vi "Read Time.vi"(8 "error in (no error)":errorcluster, 11 "ControlDragStartingMsg In":refnum<class "ControlDragStartingMsg.lvclass">) -> (0 "error out":errorcluster, 2 "Time":u32, 3 "ControlDragStartingMsg Out":refnum<class "ControlDragStartingMsg.lvclass">)   [LabVIEW 2017, in "ActorEvents.lvlib" / "ControlDragStartingMsg.lvclass"]
uses:
  ControlDragStartingMsg.lvclass
  ControlDragStartingMsg.lvclass/ControlDragStartingMsg.ctl
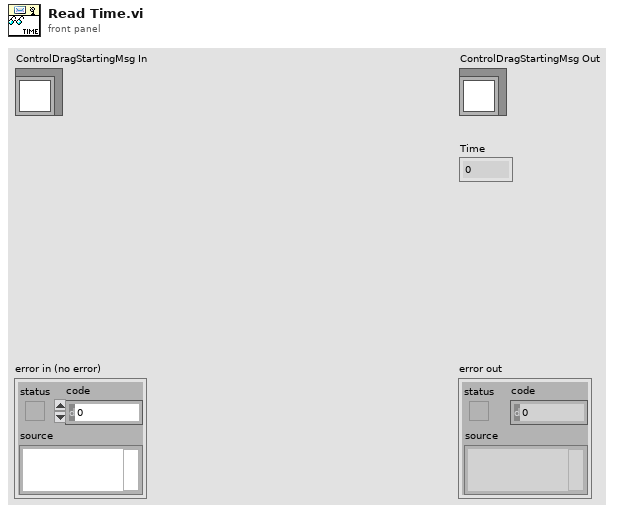
[diagram p1: front panel]
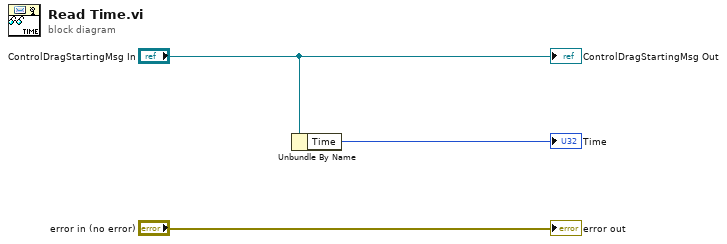
[diagram p0: block diagram]
diagram:
  n1 = Unbundle By Name("ControlDragStartingMsg In") -> ("Time"=→"Time":u32)
  "error out" <- "error in (no error)"
  "ControlDragStartingMsg Out" <- "ControlDragStartingMsg In"
